vi "SubVI_Save_Testing_Data.vi"(6 "Max_limit":i32, 8 "error in (no error)":errorcluster, 10 "Resulting Folder Path":path, 11 "Downsampled EEG In":T1) -> (0 "error out":errorcluster)   [LabVIEW 2020]
uses:
  <extravilib>/ChannelInstances/Stream-a[.](dbl)/)Channel.ctl
  <extravilib>/ChannelInstances/Stream-a[.](dbl)/EndpointRead.vi
  Global 1.vi
  <extravilib>/ChannelInstances/Stream-a[.](dbl)/)Channel.vi
  <resource>/ChannelSupport/_ChannelSupport/WaitIfNeeded.vi
  <extravilib>/ChannelInstances/Stream-a[.](dbl).lvlib
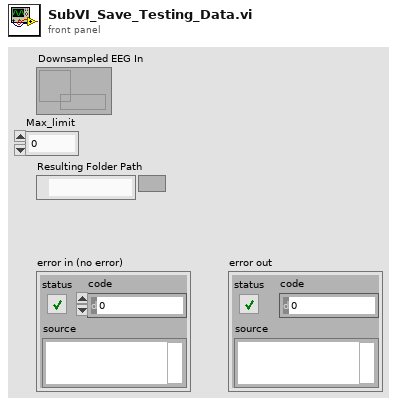
[diagram p1: front panel]
types:
  T1 = typedef "Stream-a[.](dbl).lvlib/)Channel.ctl" = refnum<queue>
  T2 = enum16{"open", "open or create", "create or replace", "create", "open (read-only)"}
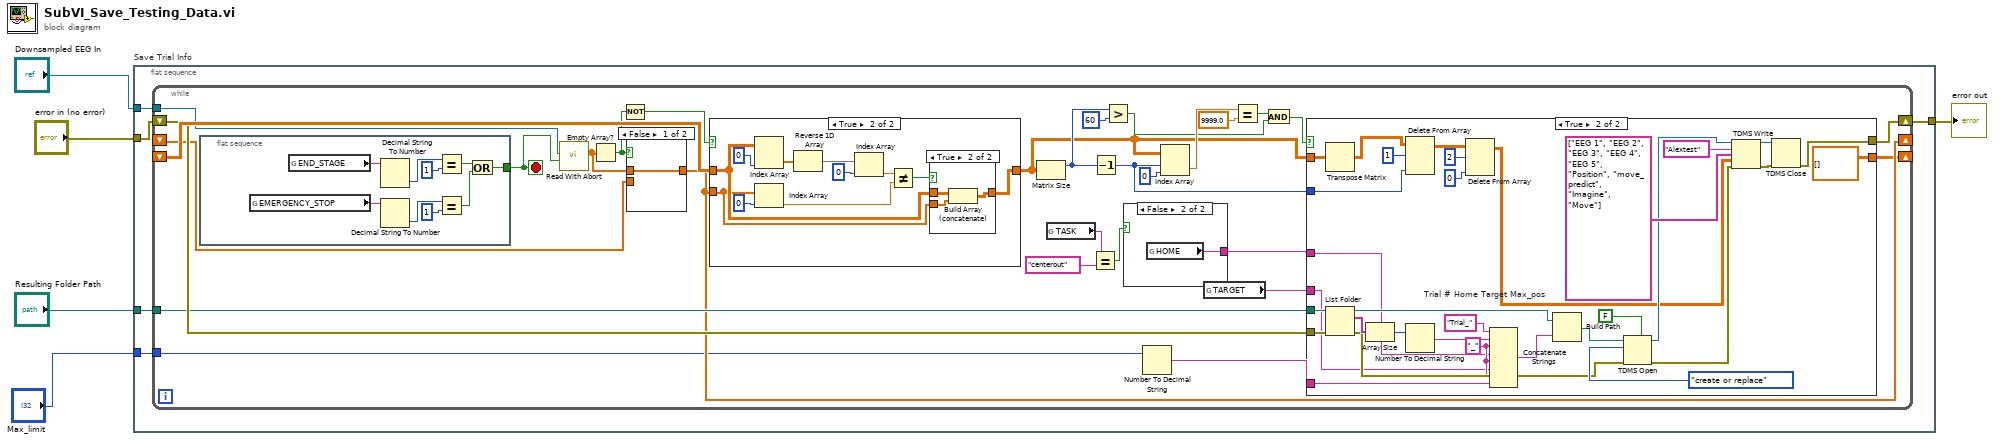
[diagram p0: block diagram]
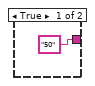
[diagram p2: hidden frame]
diagram:
  n1 = flat-sequence "Save Trial Info" {
    tunnel: "error in (no error)" -> [w10]
    tunnel: "Resulting Folder Path" -> [w9]
    tunnel: "Downsampled EEG In" -> [w8]
    tunnel: [w7] -> w4
    tunnel: "Max_limit" -> [w6]
    frame #0 {
      n2 = while {
        shift-right: [w18] -> _
        shift-left: _ -> [w39]
        tunnel: w8 -> [w38]
        shift-right: [w36] -> w7
        shift-left: w10 -> [w37]
        tunnel: w9 -> [w35]
        shift-right: [w32] -> _
        shift-left: _ -> [w33]
        tunnel: w6 -> [w16]
        stop <- w31 stop-if-true
        n3 = flat-sequence {
          tunnel: [w76] -> w31
          frame #0 {
            n4 = global read "Global 1.vi" "EMERGENCY_STOP"() -> (w79:string)
            n5 = global read "Global 1.vi" "END_STAGE"() -> (w84:string)
            n6 = Decimal String To Number(string=w84) -> (number=w83:i32)  [unwired: 2 in, 1 out]
            n7 = Decimal String To Number(string=w79) -> (number=w81:i32)  [unwired: 2 in, 1 out]
            n8 = Equal?(x=w83, y=1) -> (x = y?=w77:bool)
            n9 = Equal?(x=w81, y=1) -> (x = y?=w78:bool)
            n10 = Or(x=w77, y=w78) -> (x .or. y?=w76:bool)
          }
        }
        n11 = call <extravilib>:"Read With Abort.vi"("abort"=w31, "channel"=w38) -> ("element"=w34:dbl[])  [unwired: 4 in, 5 out]
        n12 = Empty Array?(array=w34) -> (empty?=w30:bool)
        n13 = Not(x=w30) -> (.not. x?=w29:bool)
        n14 = case shown="False" w30 {
          tunnel: w34 -> [w85 _]
          tunnel: [w85 w86] -> w32
          tunnel: w33 -> [_ w86]
          frame False {
          }
          frame True {
          }
        }
        n15 = case shown="True" w29 {
          tunnel: w39 -> [w87 w96]
          tunnel: w32 -> [_ w88]
          tunnel: [w87 w98] -> w23
          frame False {
          }
          frame True {
            n16 = Index Array(array=w96, index (col)=0 ("disabled index (row)")) -> (element=w91:dbl[])  [unwired: 1 in]
            n17 = Index Array(array=w88, index=0) -> (element=w94:dbl)
            n18 = Reverse 1D Array(array=w91) -> (reversed array=w92:dbl[])
            n19 = Index Array(array=w92, index=0 ("disabled index (row)")) -> (element=w90:dbl)
            n20 = Not Equal?(x=w90, y=w94) -> (x != y?=w97:bool)
            n21 = case shown="True" w97 {
              tunnel: w96 -> [w99 w102]
              tunnel: [w99 w101] -> w98
              tunnel: w88 -> [_ w100]
              frame False {
              }
              frame True {
                n22 = Build Array (concatenate)(w102, w100) -> (w101:dbl[][])
              }
            }
          }
        }
        n23 = Matrix Size(0:w23) -> (1:w27:i32)  [unwired: 1 out]
        n24 = global read "Global 1.vi" "TASK"() -> (w14:string)
        n25 = Equal?(x=w14, y="centerout") -> (x = y?=w12:bool)
        n26 = Decrement(x=w27) -> (x-1=w21:i32)
        n27 = Greater?(x=w27, y=60) -> (0:w19:bool)
        n28 = case shown="False" w12 {
          tunnel: ["50" ("y") w41] -> w11
          frame True {
          }
          frame False, Default {
            n29 = global read "Global 1.vi" "HOME"() -> (w41:string)
          }
        }
        n30 = Number To Decimal String(number=w16) -> (decimal integer string=w17:string)  [unwired: 1 in]
        n31 = Index Array(array=w23, index (row)=w21, index (col)=0 ("disabled index (col)")) -> (element=w25:dbl)
        n32 = global read "Global 1.vi" "TARGET"() -> (w15:string)
        n33 = Equal?(x=w25, y=9999.0) -> (x = y?=w20:bool)
        n34 = And(x=w20, y=w19) -> (x .and. y?=w22:bool)
        n35 = case shown="True" w22 {
          tunnel: w23 -> [w42 w57]
          tunnel: w37 -> [w43 w59]
          tunnel: [w43 w58] -> w36
          tunnel: w35 -> [_ w60]
          tunnel: w21 -> [_ w51]
          tunnel: [w42 dbl[][] []] -> w18
          tunnel: w17 -> [_ w46]
          tunnel: w15 -> [_ w45]
          tunnel: w11 -> [_ w44]
          frame False {
          }
          frame True {
            w47 = "_" ("string")
            n36 = Transpose Matrix(1:w57) -> (0:w50:dbl[][])
            n37 = List Folder(path=w60, error in=w59) -> (path out=w56:path, filenames=w65:string[], error out=w63:errorcluster)  [unwired: 2 in, 1 out]
            n38 = Array Size(array=w65) -> (size(s)=w66:i32)
            n39 = Delete From Array(array=w50, length=1, index (col)=w51) -> (array with subset deleted=w49:dbl[][])  [unwired: 1 in, 1 out]
            n40 = Number To Decimal String(number=w66) -> (decimal integer string=w64:string)  [unwired: 1 in]
            n41 = Delete From Array(array=w49, length=2, index (col)=0 ("disabled index (col)")) -> (array with subset deleted=w53:dbl[][])  [unwired: 1 in, 1 out]
            n42 = Concatenate Strings "Trial # Home Target Max_pos"("Trial_" ("string"), w64, w47, w44, w47, w45, w47, w46) -> (w75:string)
            n43 = Build Path(base path=w56, name or relative path=w75) -> (appended path=w73:path)
            n44 = TDMS Open(5:FALSE ("create index file? (T)"), 8:w63, 10:T2."create or replace" ("operation (0:open)"), 11:w73) -> (0:w62:errorcluster, 3:w69:refnum<k34>)  [unwired: 3 in]
            n45 = TDMS Write(0:w69, 5:"Alextest" ("group name in (Untitled)"), 7:string[] ["EEG 1", "EEG 2", "EEG 3", "EEG 4", "EEG 5", "Position", "move_predict", "Imagine", "Move"] ("channel name(s) in (Untitled)"), 9:w53, 11:w62) -> (4:w72:refnum<k34>, 15:w61:errorcluster)  [unwired: 1 in, 2 out]
            n46 = TDMS Close(8:w61, 11:w72) -> (0:w58:errorcluster)  [unwired: 1 out]
          }
        }
      }
    }
  }
  "error out" <- w4
